vi "usrp set dboard eeprom.vi"(6 "mboard":u64, 7 "slot":string, 8 "error in (no error)":errorcluster, 9 "unit":string, 10 "db_eeprom":u64, 11 "h":u64) -> (0 "error out":errorcluster, 3 "function return":u32(ring))   [LabVIEW 2023, in "uhd.lvlib"]
doc: "UHD_API uhd_error uhd_usrp_set_dboard_eeprom(uhd_usrp_handle h,\n uhd_dboard_eeprom_handle db_eeprom,\n const char* unit,\n const char* slot,\n size_t mboard);"
uses:
  <userlib>/uhd/uhd.lvlib
  <userlib>/uhd/uhd.dll
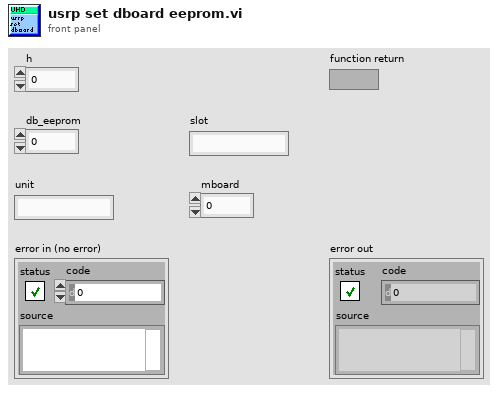
[diagram p1: front panel]
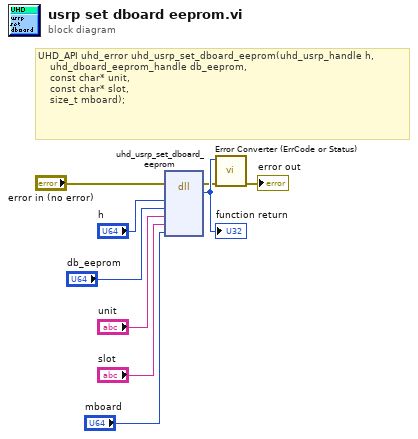
[diagram p0: block diagram]
diagram:
  # "UHD_API uhd_error uhd_usrp_set_dboard_eeprom(uhd_usrp_handle h,\n    uhd_dboard_eeprom_handle db_eeprom,\n    const char* unit,\n    const char* slot,\n    size_t mboard);"
  n1 = dll-call lib="C:/Program Files/National Instruments/LabVIEW 2023/user.lib/uhd/uhd.*" fn="uhd_usrp_set_dboard_eeprom"(error in="error in (no error)", "h"="h", "db_eeprom"="db_eeprom", "unit"="unit", "slot"="slot", "mboard"="mboard") -> (error out=w2:errorcluster, w9:u32)  [unwired: 7 in, 1 out]
  "function return" <- w9
  n2 = call <userlib>:"Error Converter (ErrCode or Status).vi"("error in (no error)"=w2, "error code"=w9) -> ("error out"=→"error out":errorcluster)  [unwired: 9 in]
